vi "Write Gain Selection.vi"(8 "error in (no error)":errorcluster, 10 "Gain Values":T1, 11 "LINX-ADS1X15 in":refnum<class "LINX-ADS1256.lvclass">) -> (0 "error out":errorcluster, 3 "LINX-ADS1X15 out":refnum<class "LINX-ADS1256.lvclass">)   [LabVIEW 2020, in "LINX-ADS1256.lvclass"]
uses:
  LINX-ADS1256.lvclass
  Programmable Gain Selection.ctl
  LINX-ADS1256.lvclass/LINX-ADS1256.ctl
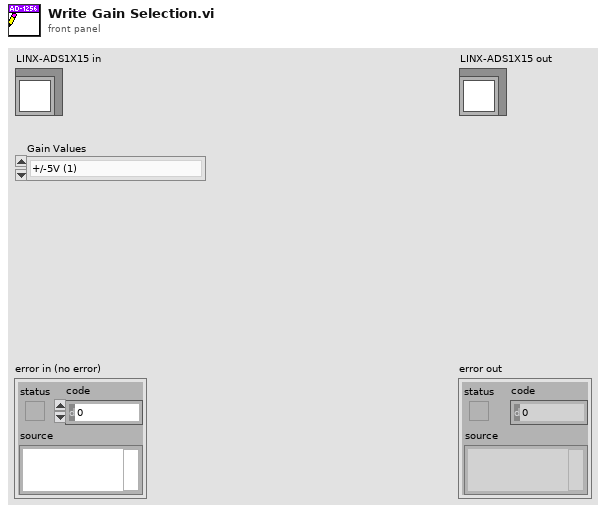
[diagram p1: front panel]
types:
  T1 = typedef "LINX-ADS1256.lvclass/Programmable Gain Selection.ctl" = enum16{"+/-5V (1)", "+/-2.5V (2)", "+/-1.25V (4)", "+/-0.625V (8)", "+/-312.5mV (16)", "+/-156.25mV (32)", "+/-78.125mV (64)"}
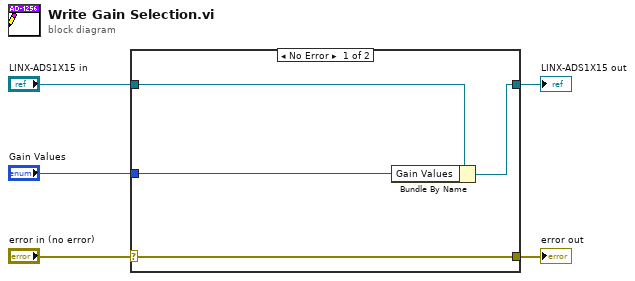
[diagram p0: block diagram]
diagram:
  n1 = case shown="No Error" "error in (no error)" {
    selector: "error in (no error)" -> [w9 w10]
    tunnel: [w9 w10] -> w4
    tunnel: [w7 w11] -> w2
    tunnel: "LINX-ADS1X15 in" -> [w8 w11]
    tunnel: "Gain Values" -> [w6 _]
    frame No Error {
      n2 = Bundle By Name(cluster=w8, "Gain Values"=w6) -> (w7:refnum<class "LINX-ADS1256.lvclass">)
    }
    frame Error {
    }
  }
  "error out" <- w4
  "LINX-ADS1X15 out" <- w2
